vi "prova.vi"(1 "filter index":u8(ring) items=["ch_BFP", "ch_Cerulean", "ch_GFP", "ch_mOrange", "ch_mCherry", "ch_mNeptune"]) -> ()   [LabVIEW 2017]
panel:
  out "decimal integer string":string
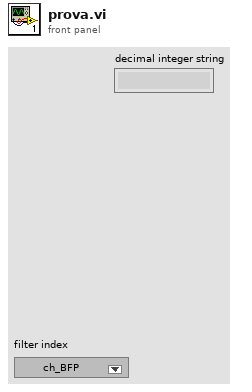
[diagram p1: front panel]
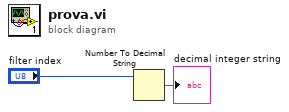
[diagram p0: block diagram]
diagram:
  n1 = Number To Decimal String(number="filter index") -> (decimal integer string=→"decimal integer string":string)  [unwired: 1 in]
